vi "Get port Status.vi"(8 "error in (no error)":errorcluster, 10 "Puerto":dbl, 11 "Arduino in":refnum<class "Arduino.lvclass">) -> (0 "error out":errorcluster, 3 "Arduino out":refnum<class "Arduino.lvclass">)   [LabVIEW 2020, in "Arduino.lvclass"]
uses:
  Arduino.lvclass
  047f6691-8673-4972-af87-69d58803e37a.vi
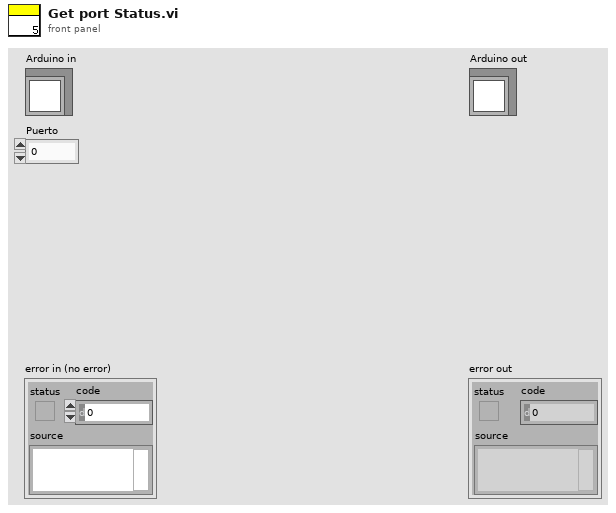
[diagram p1: front panel]
types:
  T1 = typedef "Serial Device.lvclass/serial device brand.ctl" = string
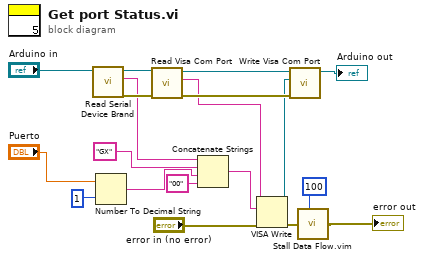
[diagram p0: block diagram]
diagram:
  n1 = call-dynamic "Read Serial Device Brand.vi"("Serial Device in"="Arduino in") -> ("error out"=w14:errorcluster, "Serial Device Brand"=w7:T1, "Serial Device out"=w18:refnum<class "Arduino.lvclass">)  [unwired: 8 in]
  n2 = Number To Decimal String(number="Puerto", width (-)=i16 1) -> (decimal integer string=w5:string)
  n3 = call-dynamic "Read Visa Com Port.vi"("error in (no error)"=w14, "Serial Device in"=w18) -> ("error out"=w15:errorcluster, "Visa Com Port"=w9:string, "Serial Device out"=w17:refnum<class "Arduino.lvclass">)  [unwired: 7 in]
  n4 = Concatenate Strings(w7, "GX" ("string"), w5, "00" ("string")) -> (w10:string)
  n5 = VISA Write(VISA resource name=w9, write buffer=w10, error in (no error)="error in (no error)") -> (VISA resource name out=w8:refnum<visa-resource-name>, error out=w3:errorcluster)  [unwired: 1 out]
  n6 = call-dynamic "Write Visa Com Port.vi"("error in (no error)"=w15, "Visa Com Port"=w8, "Serial Device in"=w17) -> ("Serial Device out"=→"Arduino out":refnum<class "Arduino.lvclass">)  [unwired: 7 in, 1 out]
  n7 = call "Stall Data Flow.vim"("value in"=w3, "milliseconds to wait"=u32 100) -> ("value out"=→"error out":errorcluster)  [unwired: 1 out]
